vi "DeserializeFaceEncoding.vi"(8 "error in (no error)":errorcluster, 10 "BinaryEncoding":u8[](array[numeric])) -> (0 "error out":errorcluster, 3 "FaceEncoding":refnum<k24>)   [LabVIEW 2020, in "FaceRecognitionDotNet.lvlib" / "FaceRecognition.lvclass"]
uses:
  FaceRecognition.lvclass
  dll/FaceRecognitionDotNet.dll
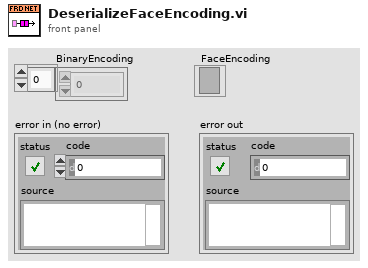
[diagram p1: front panel]
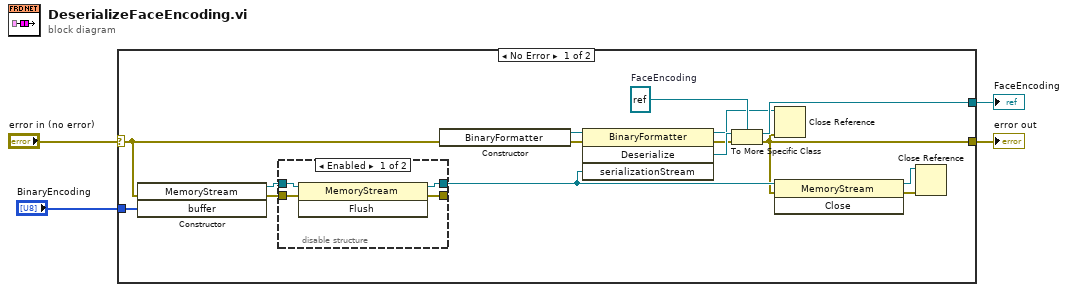
[diagram p0: block diagram]
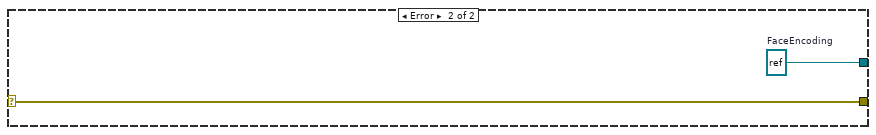
[diagram p3: hidden frame]
diagram:
  n1 = case shown="No Error" "error in (no error)" {
    selector: "error in (no error)" -> [w7 w26]
    tunnel: "BinaryEncoding" -> [w19 _]
    tunnel: [w18 w27] -> w3
    tunnel: [w5 w26] -> w2
    frame No Error {
      w16 = refnum<k24> refnum  # FaceEncoding
      n2 = constructor class="MemoryStream"(error in=w7, "buffer"=w19) -> (reference out=w14:refnum<k24>, error out=w15:errorcluster)  [unwired: 2 in, 2 out]
      n3 = disable-structure shown="Enabled" {
        disable-tunnel: [w23 w24] -> _
        disable-tunnel: w15 -> [w22 w24]
        disable-tunnel: [w21 w25] -> w11
        disable-tunnel: w14 -> [w20 w25]
        frame Enabled {
          n4 = invoke class="MemoryStream" method="Flush"(reference=w20, error in=w22) -> (reference out=w21:refnum<k24>, error out=w23:errorcluster)  [unwired: 1 in, 1 out]
        }
        frame Disabled {
        }
      }
      n5 = constructor class="BinaryFormatter"(error in=w7) -> (reference out=w17:refnum<k24>, error out=w8:errorcluster)  [unwired: 2 in, 1 out]
      n6 = invoke class="BinaryFormatter" method="Deserialize"(reference=w17, error in=w8, "serializationStream"=w11) -> (reference out=w12:refnum<k24>, error out=w6:errorcluster, "Deserialize"=w13:refnum<k24>)  [unwired: 1 in, 1 out]
      n7 = To More Specific Class(target class=w16, reference=w13, error in=w6) -> (specific class reference=w18:refnum<k24>, error out=w5:errorcluster)
      n8 = Close Reference(reference=w12, error in (no error)=w5) -> ()  [unwired: 1 out]
      n9 = invoke class="MemoryStream" method="Close"(reference=w11, error in=w5) -> (reference out=w9:refnum<k24>, error out=w10:errorcluster)  [unwired: 1 in, 1 out]
      n10 = Close Reference(reference=w9, error in (no error)=w10) -> ()  [unwired: 1 out]
    }
    frame Error {
      w27 = refnum<k24> refnum  # FaceEncoding
    }
  }
  "error out" <- w2
  "FaceEncoding" <- w3
